vi "Get Sparse Marker Name [SM] Core.vi"(8 "error in (no error)":errorcluster, 9 "Name Buffer Size":i32 format="%.0g", 10 "Marker Index (1)":i32=1 format="%.0g", 11 "CS++Fgen in":refnum<class "CS++Fgen.lvclass">) -> (0 "error out":errorcluster, 2 "Marker Name":string, 3 "CS++Fgen out":refnum<class "CS++Fgen.lvclass">)   [LabVIEW 2015, in "CS++Fgen.lvlib" / "CS++Fgen.lvclass"]
doc: "This VI returns the repeated capability identifier for the data marker that corresponds to the one-based index that you specify. If the value that you pass for the Marker Index control is less than one or greater than the value of the data marker count, the VI returns an empty string in the Marker Name control and returns an error.\n\nNote:\n\n(1) This VI is part of the IviFgenSparseMarker [SM] extension group."
uses:
  CS++Fgen.lvclass
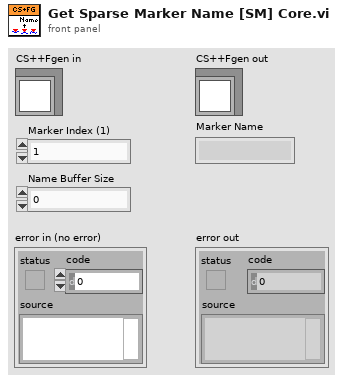
[diagram p1: front panel]
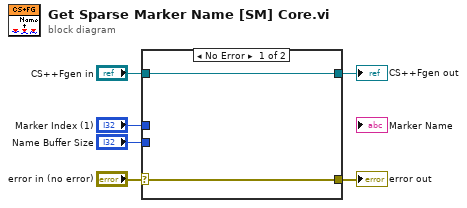
[diagram p0: block diagram]
diagram:
  n1 = case shown="No Error" "error in (no error)" {
    selector: "error in (no error)" -> [w7 w10]
    tunnel: [w7 w10] -> w5
    tunnel: [w8 w9] -> w3
    tunnel: "CS++Fgen in" -> [w8 w9]
    tunnel: "Marker Index (1)" -> [_ _]
    tunnel: "Name Buffer Size" -> [_ _]
    frame No Error {
    }
    frame Error {
    }
  }
  "error out" <- w5
  "CS++Fgen out" <- w3
